vi "Setup.vi"(8 "error in (no error)":errorcluster) -> (0 "error out":errorcluster, 3 "Bus Controller out":refnum<class "Bus Controller.lvclass">)   [LabVIEW 2020, in "Unit Tests.lvlib" / "Bus Controller.lvclass"]
uses:
  Bus Controller.lvclass
  Dependencies/Registry/Registry.lvclass/Registry.ctl
  Bus Controller.lvclass/Bus Controller.ctl
  Utilities/Simulated FPGA/FPGA Sim.lvclass
  C:/Users/MattJ/Desktop/git/bci-1553-labview-api/src/Dependencies/FPGA Interface/FPGA Interface.lvclass
  Dependencies/Registry/Registry.lvclass
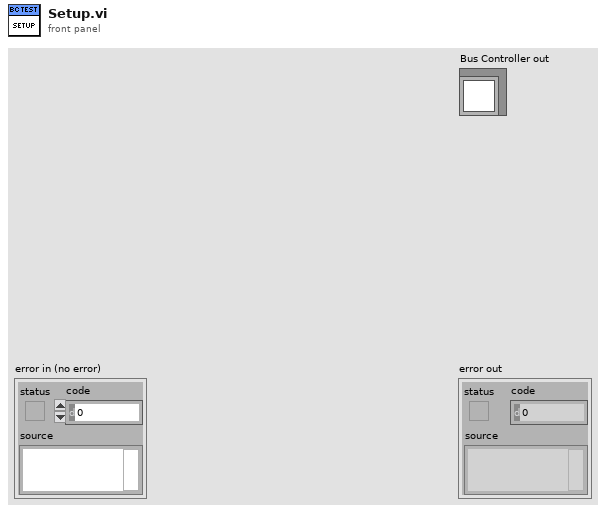
[diagram p1: front panel]
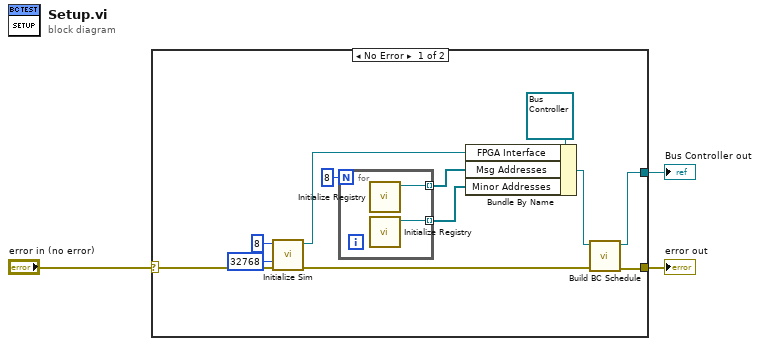
[diagram p0: block diagram]
diagram:
  n1 = case shown="No Error" "error in (no error)" {
    selector: "error in (no error)" -> [w11 w18]
    tunnel: [w8 w18] -> w2
    tunnel: [w9 _] -> w1
    frame No Error {
      n2 = call "Initialize Sim.vi"("error in (no error)"=w11, "Memory Size (32k)"=32768, "Components (8)"=8) -> ("error out"=w4:errorcluster, "FPGA Sim out"=w12:refnum<class "FPGA Sim.lvclass">)  [unwired: 7 in]
      n3 = for {
        N: 8 -> [_]
        tunnel: [w17] -> w7 mode=indexing
        tunnel: [w16] -> w6 mode=indexing
        n4 = call "Initialize Registry.vi"() -> ("Registry out"=w17:refnum<class "Registry.lvclass">)  [unwired: 10 in, 1 out]
        n5 = call "Initialize Registry.vi"() -> ("Registry out"=w16:refnum<class "Registry.lvclass">)  [unwired: 10 in, 1 out]
      }
      n6 = Bundle By Name(cluster=refnum<class "Bus Controller.lvclass"> refnum ("Bus Controller in"), "FPGA Interface"=w12, "Msg Addresses"=w7, "Minor Addresses"=w6) -> (w10:refnum<class "Bus Controller.lvclass">)
      n7 = call "Build BC Schedule.vi"("error in (no error)"=w4, "Bus Controller in"=w10) -> ("error out"=w8:errorcluster, "Bus Controller out"=w9:refnum<class "Bus Controller.lvclass">)  [unwired: 8 in]
    }
    frame Error {
    }
  }
  "error out" <- w2
  "Bus Controller out" <- w1
